vi "Prefix Array.vi"(6 "End Symbol":string, 7 "Start Symbol":string, 8 "error in (no error)":errorcluster, 10 "Array":string[](array[string]), 11 "JSON Serializer in":refnum<class "JSON Serializer.lvclass">) -> (0 "error out":errorcluster, 2 "String":string, 3 "JSON Serializer out":refnum<class "JSON Serializer.lvclass">)   [LabVIEW 2019, in "JKI JSON Serialization.lvlib" / "JSON Serializer.lvclass"]
doc: "JKI JSON 1.1.10.37\nTomi Maila - JKI\nCopyright (c) 2017, JKI"
uses:
  JSON Serializer.lvclass
  JSON Serializer.lvclass/JSON Serializer.ctl
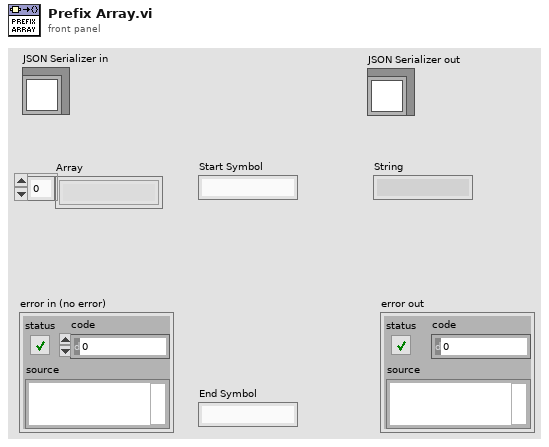
[diagram p1: front panel]
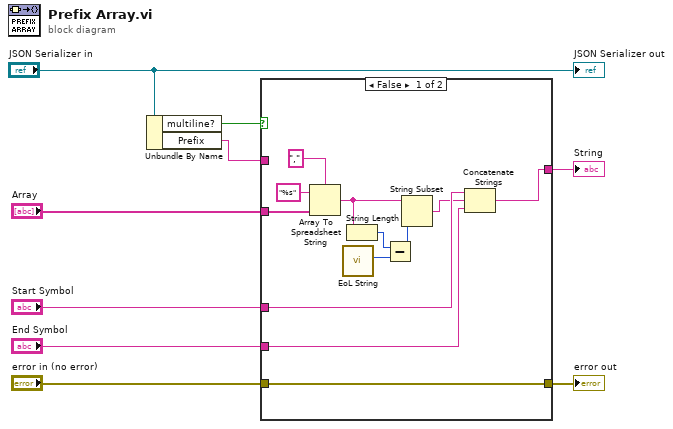
[diagram p0: block diagram]
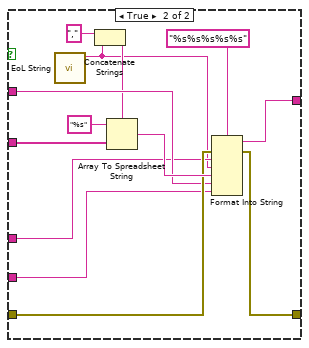
[diagram p2: hidden frame]
diagram:
  n1 = Unbundle By Name("JSON Serializer in") -> ("multiline?"=w2:bool, "Prefix"=w1:string)
  n2 = case shown="False" w2 {
    tunnel: "error in (no error)" -> [w15 w33]
    tunnel: [w15 w32] -> w8
    tunnel: [w16 w31] -> w7
    tunnel: "Array" -> [w19 w29]
    tunnel: w1 -> [_ w27]
    tunnel: "Start Symbol" -> [w18 w23]
    tunnel: "End Symbol" -> [w17 w26]
    frame False {
      n3 = Array To Spreadsheet String(delimiter (Tab)=",", array=w19, 3:"%s" ("format string")) -> (spreadsheet string=w14:string)
      n4 = call "EoL String.vi"() -> ("EoL String Length"=w12:i32)  [unwired: 10 in, 1 out]
      n5 = String Length(string=w14) -> (length=w11:i32)
      n6 = Subtract(x=w11, y=w12) -> (x-y=w10:i32)
      n7 = String Subset(string=w14, length (rest)=w10) -> (substring=w13:string)  [unwired: 1 in]
      n8 = Concatenate Strings(w18, w13, w17) -> (w16:string)
    }
    frame True {
      n9 = call "EoL String.vi"() -> ("EoL String"=w22:string)  [unwired: 10 in, 1 out]
      n10 = Concatenate Strings("," ("delimiter (Tab)"), w22) -> (w24:string)
      n11 = Array To Spreadsheet String(delimiter (Tab)=w24, array=w29, 3:"%s" ("format string")) -> (spreadsheet string=w34:string)
      n12 = Format Into String(format string="%s%s%s%s%s", error in=w33, w23, w22, w34, w27, w26) -> (resulting string=w31:string, error out=w32:errorcluster)  [unwired: 1 in]
    }
  }
  "error out" <- w8
  "String" <- w7
  "JSON Serializer out" <- "JSON Serializer in"
